vi "util_change_in_read.vi"(7 "references":T1, 8 "error in (no error)":errorcluster, 10 "timeout":i32) -> (0 "error out":errorcluster, 2 "data":variant, 3 "change?":bool)   [LabVIEW 2015, in "lv-recipe-machine.lvlib"]
uses:
  lv-recipe-machine.lvlib
  public/_controls/references.ctl
  _controls/input.ctl
  _controls/input_command.ctl
  _controls/output.ctl
  _controls/data.ctl
  public/_controls/configuration.ctl
  _controls/recipe_data.ctl
  public/_controls/mode.ctl
  public/_controls/manual_state.ctl
  public/_controls/automatic_state.ctl
  public/_controls/recipe_step.ctl
  <userlib>/antonio-alexander/lv-waitgroup/public/_controls/api_waitgroup.ctl
  public/_controls/transition.ctl
  public/_controls/change.ctl
  public/_controls/status.ctl
  <userlib>/antonio-alexander/lv-waitgroup/lv-waitgroup.lvlib
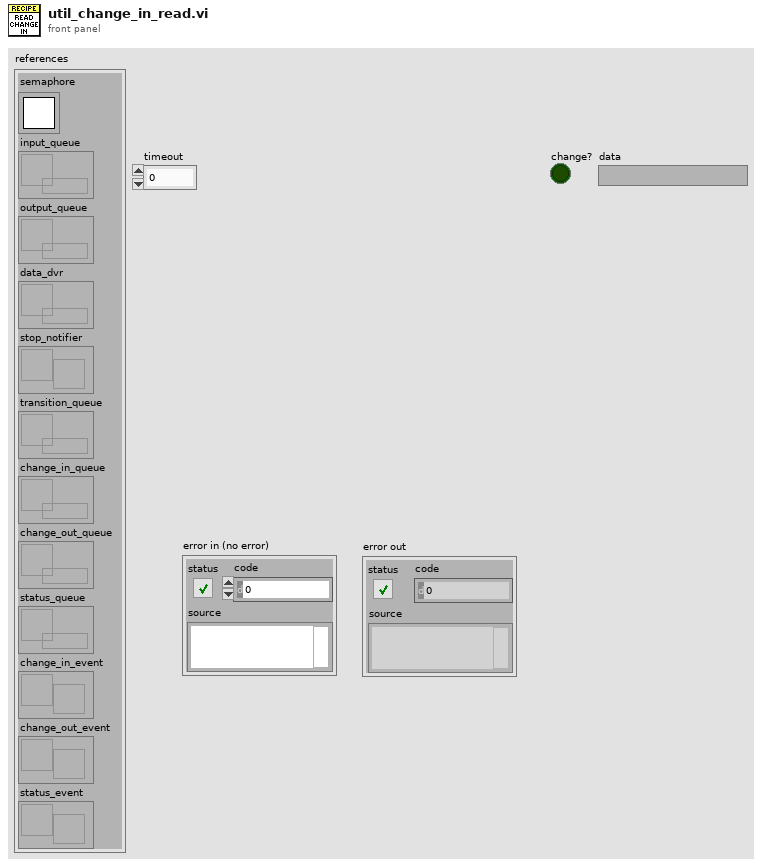
[diagram p1: front panel]
types:
  T1 = typedef "lv-recipe-machine.lvlib/references.ctl" = cluster{"semaphore":T2, "input_queue":refnum<queue>, "output_queue":refnum<queue>, "data_dvr":refnum<data-value>, "stop_notifier":refnum<notifier>, "transition_queue":refnum<queue>, "change_in_queue":refnum<queue>, "change_out_queue":refnum<queue>, "status_queue":refnum<queue>, "change_in_event":refnum<user-event>, "change_out_event":refnum<user-event>, "status_event":refnum<user-event>}
  T2 = typedef "Semaphore RefNum" = refnum<k1>
  T3 = typedef "lv-recipe-machine.lvlib/change.ctl" = cluster{"changed":bool, "data":variant}
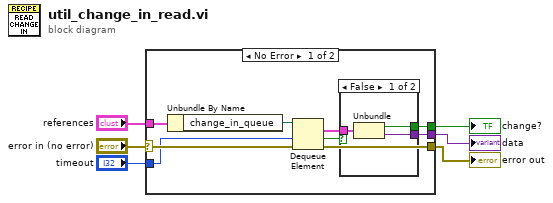
[diagram p0: block diagram]
diagram:
  n1 = case shown="No Error" "error in (no error)" {
    selector: "error in (no error)" -> [w8 w19]
    tunnel: [w13 w19] -> w5
    tunnel: "references" -> [w15 _]
    tunnel: "timeout" -> [w7 _]
    tunnel: [w10 _] -> w2
    tunnel: [w9 _] -> w1
    frame No Error {
      n2 = Unbundle By Name(w15) -> ("change_in_queue"=w14:refnum<queue>)
      n3 = Dequeue Element(queue=w14, timeout in ms (-1)=w7, error in (no error)=w8) -> (element=w11:T3, timed out?=w12:bool, error out=w13:errorcluster)  [unwired: 1 out]
      n4 = case shown="False" w12 {
        tunnel: w11 -> [w18 _]
        tunnel: [w17 _] -> w10
        tunnel: [w16 _] -> w9
        frame False {
          n5 = Unbundle(w18) -> ("changed"=w17:bool, "data"=w16:variant)
        }
        frame True {
        }
      }
    }
    frame Error {
    }
  }
  "error out" <- w5
  "change?" <- w2
  "data" <- w1
